vi "API - DIO - Set Digital Output.vi"(8 "error in":errorcluster, 9 "State":bool, 10 "Channel Number":i32, 11 "DAQiFi Device Properties In":T1) -> (0 "error out":errorcluster, 3 "DAQiFi Device Properties Out":T1)   [LabVIEW 2021]
doc: "Set the state of a digital output. Before setting the state, the channel must be enabled as a digital output."
uses:
  TypeDefs/TypeDef - Cluster of DAQiFi Device Properties.ctl
  TypeDefs/Enum - Connection Type.ctl
  TCP - Write and Read a Synchronous Message.vi
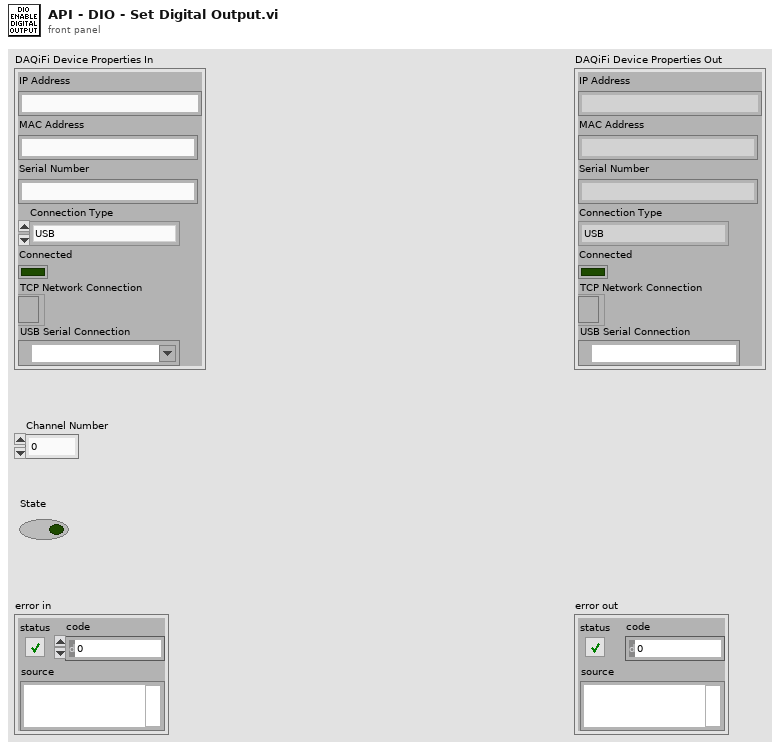
[diagram p1: front panel]
types:
  T1 = typedef "TypeDef - Cluster of DAQiFi Device Properties.ctl" = cluster{"IP Address":string, "MAC Address":string, "Serial Number":string, "Connection Type":T2, "Connected":bool, "TCP Network Connection":refnum<k5>, "USB Serial Connection":refnum<visa-resource-name>}
  T2 = typedef "Enum - Connection Type.ctl" = enum16{"USB", "TCP"}
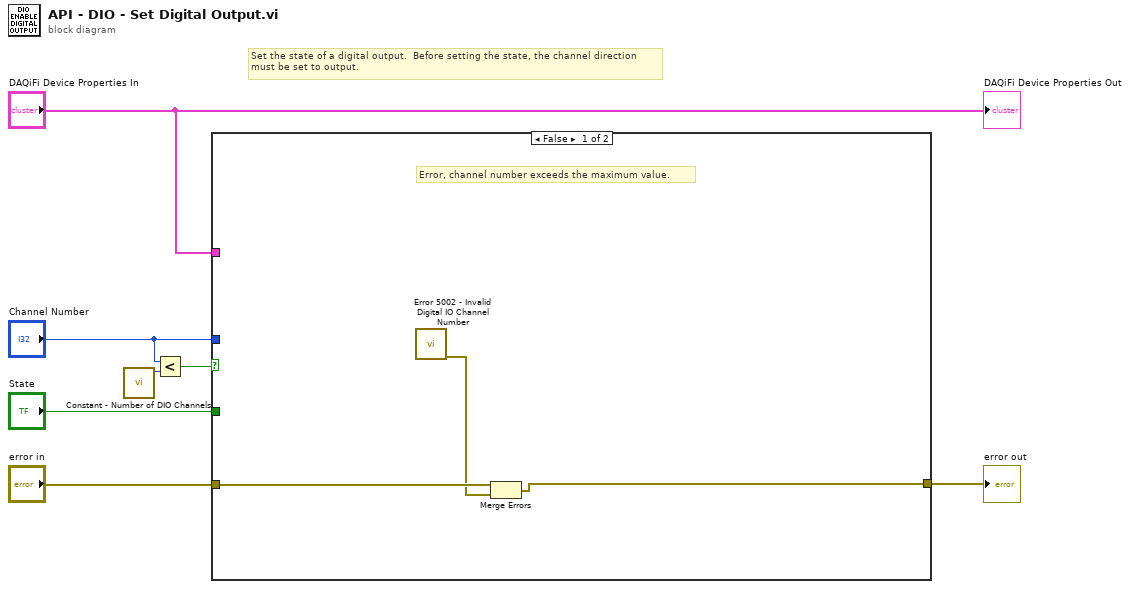
[diagram p0: block diagram]
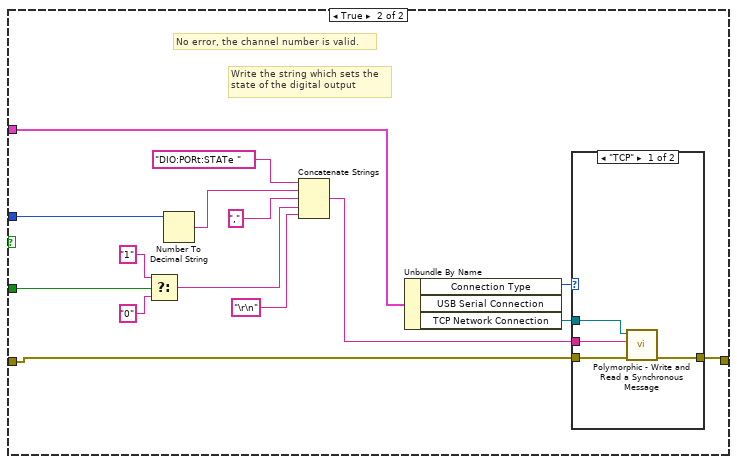
[diagram p2: hidden frame]
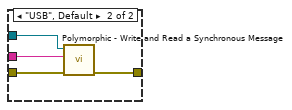
[diagram p3: hidden frame]
diagram:
  # "Set the state of a digital output.  Before setting the state, the channel direction\nmust be set to output."
  n1 = call "Constant - Number of DIO Channels.vi"() -> ("Maximum Channel"=w3:i32)  [unwired: 11 in]
  n2 = Less?(x="Channel Number", y=w3) -> (x < y?=w2:bool)
  n3 = case shown="False" w2 {
    tunnel: "error in" -> [w10 w14]
    tunnel: [w9 w13] -> w6
    tunnel: "State" -> [_ w22]
    tunnel: "Channel Number" -> [_ w17]
    tunnel: "DAQiFi Device Properties In" -> [_ w16]
    frame False {
      # "Error, channel number exceeds the maximum value."
      n4 = call "Error 5002 - Invalid Digital IO Channel Number.vi"() -> ("error out"=w8:errorcluster)  [unwired: 11 in]
      n5 = Merge Errors(w10, w8) -> (w9:errorcluster)
    }
    frame True {
      # "Write the string which sets the\nstate of the digital output"
      # "No error, the channel number is valid."
      n6 = Select(t="1", s=w22, f="0") -> (s? t:f=w19:string)
      n7 = Number To Decimal String(number=w17) -> (decimal integer string=w24:string)  [unwired: 1 in]
      n8 = Concatenate Strings("DIO:PORt:STATe " ("Message to Send"), w24, "," ("string"), w19, "\r\n" ("string")) -> (w11:string)
      n9 = Unbundle By Name(w16) -> ("Connection Type"=w15:T2, "TCP Network Connection"=w12:refnum<k5>)  [unwired: 1 out]
      n10 = case shown="\"TCP\"" w15 {
        tunnel: w14 -> [w29 w33]
        tunnel: [w28 w32] -> w13
        tunnel: w12 -> [w27 w31]
        tunnel: w11 -> [w26 w30]
        frame "TCP" {
          n11 = call-poly "Polymorphic - Write and Read a Synchronous Message.vi"("error in"=w29, "Message to Send"=w26, "TCP Network Connection in"=w27) -> ("error out"=w28:errorcluster)  [unwired: 6 in, 2 out]
        }
        frame "USB", Default {
          n12 = call-poly "Polymorphic - Write and Read a Synchronous Message.vi"("error in"=w33, "Message to Send"=w30, "TCP Network Connection in"=w31) -> ("error out"=w32:errorcluster)  [unwired: 6 in, 2 out]
        }
      }
    }
  }
  "error out" <- w6
  "DAQiFi Device Properties Out" <- "DAQiFi Device Properties In"
